vi "Filter Error Codes__ogtk.vi"   [LabVIEW 2023, in "openg_error.lvlib"]
doc: "Filters <b>Error In</b> if matches <b>Error Code to Filter</b>. An <b>Upstream Error</b> can be optionally merged with the resulting filtered error."
uses:
  openg_error.lvlib
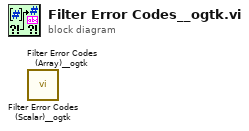
[diagram p0: block diagram]
diagram:
  n1 = call "Filter Error Codes (Scalar)__ogtk.vi"() -> ()  [unwired: 9 in, 3 out]
  n2 = call "Filter Error Codes (Array)__ogtk.vi"() -> ()  [unwired: 9 in, 3 out]
